vi "Generate Unique Header.vi"(8 "error in (no error)":errorcluster, 11 "MC Data in":refnum<class "MC Data.lvclass">) -> (0 "error out":errorcluster, 2 "Header":string[](array[string]), 3 "MC Data out":refnum<class "MC Data.lvclass">)   [LabVIEW 2014, in "Alicat Lib.lvlib" / "MC Data.lvclass"]
uses:
  MC Data.lvclass
  reusable/Data/Data.lvclass/Data.ctl
  reusable/Data/Read Data ID.vi
  Alicat Data.lvclass
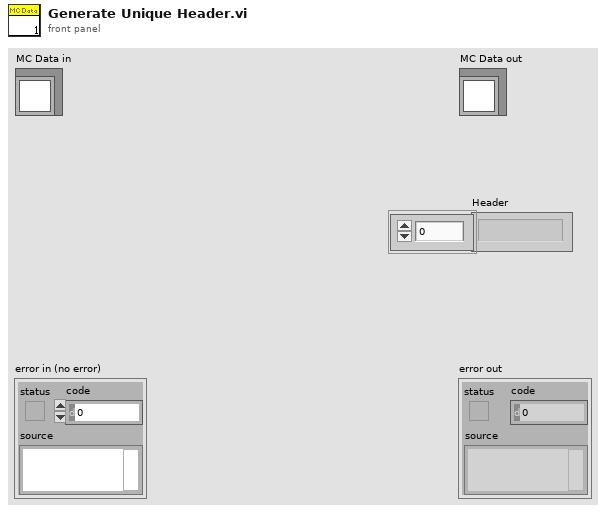
[diagram p1: front panel]
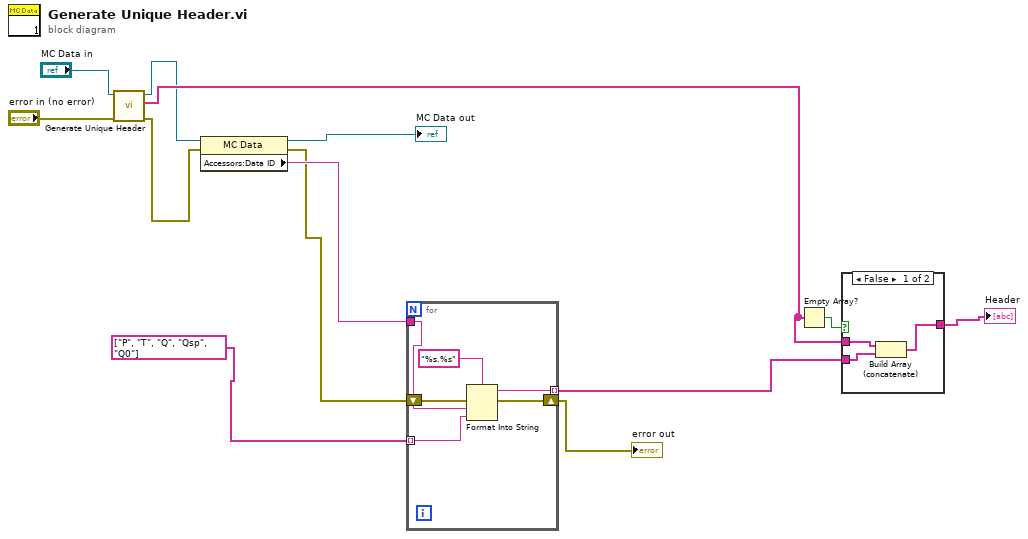
[diagram p0: block diagram]
diagram:
  n1 = call-parent "Generate Unique Header.vi"("error in"="error in (no error)", "Alicat Data in"="MC Data in") -> ("error out"=w2:errorcluster, "Header"=w10:string[], "Alicat Data out"=w5:refnum<class "MC Data.lvclass">)  [unwired: 7 in]
  n2 = property class="MC Data"(reference=w5, error in=w2) -> (reference out=→"MC Data out":refnum<class "MC Data.lvclass">, error out=w1:errorcluster, "Accessors:Data ID"=w3:string)
  n3 = for {
    tunnel: string[] ["P", "T", "Q", "Qsp", "Q0"] -> [w17] mode=indexing
    tunnel: w3 -> [w18]
    tunnel: [w16] -> w7 mode=indexing
    shift-right: [w14] -> w6
    shift-left: w1 -> [w15]
    n4 = Format Into String(format string="%s.%s", error in=w15, w18, w17) -> (resulting string=w16:string, error out=w14:errorcluster)  [unwired: 1 in]
  }
  "error out" <- w6
  n5 = Empty Array?(array=w10) -> (empty?=w11:bool)
  n6 = case shown="False" w11 {
    tunnel: w7 -> [w22 w23]
    tunnel: [w20 w23] -> w9
    tunnel: w10 -> [w21 _]
    frame False {
      n7 = Build Array (concatenate)(w21, w22) -> (w20:string[])
    }
    frame True {
    }
  }
  "Header" <- w9
